vi "MPS_ErrorMessage.vi"(11 "error code (no error:0)":i32=5001) -> (0 "error out":errorcluster, 1 "message":string=" INSTRUCTIONS:\r\rNormal Use:  When using subVIs that incorporate the error in/error out (or error I/O) structure, place this handler where you want to inform the user of an error, typically at the end of the I/O data path, as the last action of the program.  If the error in error? is ERROR, the handler creates a message describing the error and its source.  If the type of dialog = 1 (default), the message is displayed to the user, who can only acknowedge it.  If the type = 2, the user can acknowledge the message or abort execution; aborting a program with active I/O is not recommended.  If the type = 0, no message is displayed; this is used to process the error programmatically, and the error out cluster elements are wired to individual terminals for that reason.  \r\rOther Use:\n\r\nlocal testing.  To test the error code of a subVI or function that does not have the error I/O structure, you can wire its error code and a source string to the local error code and error source inputs.  If error in error? indicates no error and error code is not equal to 0, the local code and source are substituted for the error in values, and error? is set TRUE (ERROR).", 3 "code out":i32 format="%0.0f", 5 "error?":bool)   [LabVIEW 2021]
uses:
  <vilib>/Utility/error.llb/DialogType.ctl
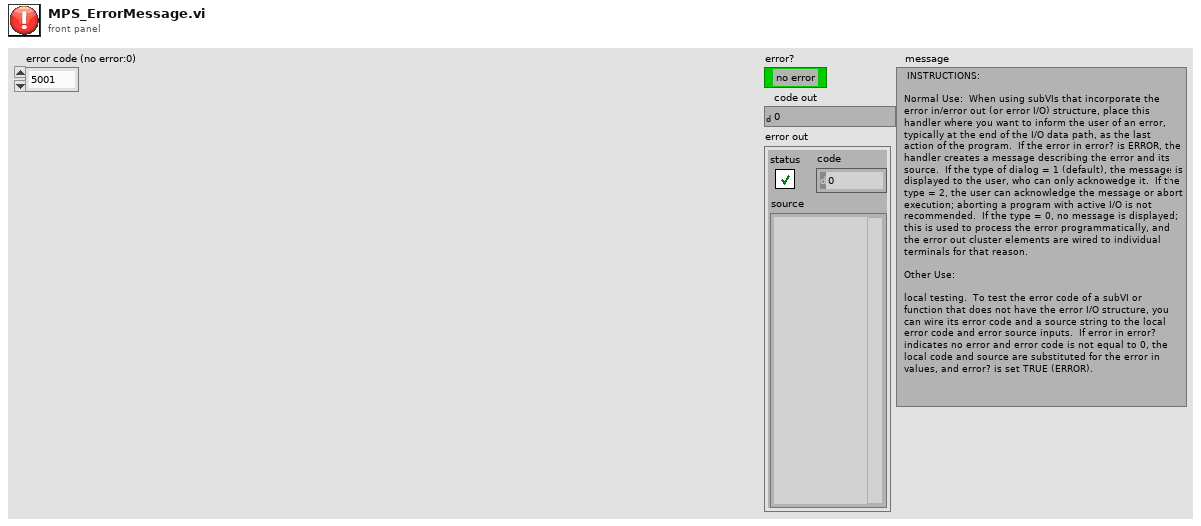
[diagram p1: front panel]
types:
  T1 = typedef "DialogType.ctl" = u16
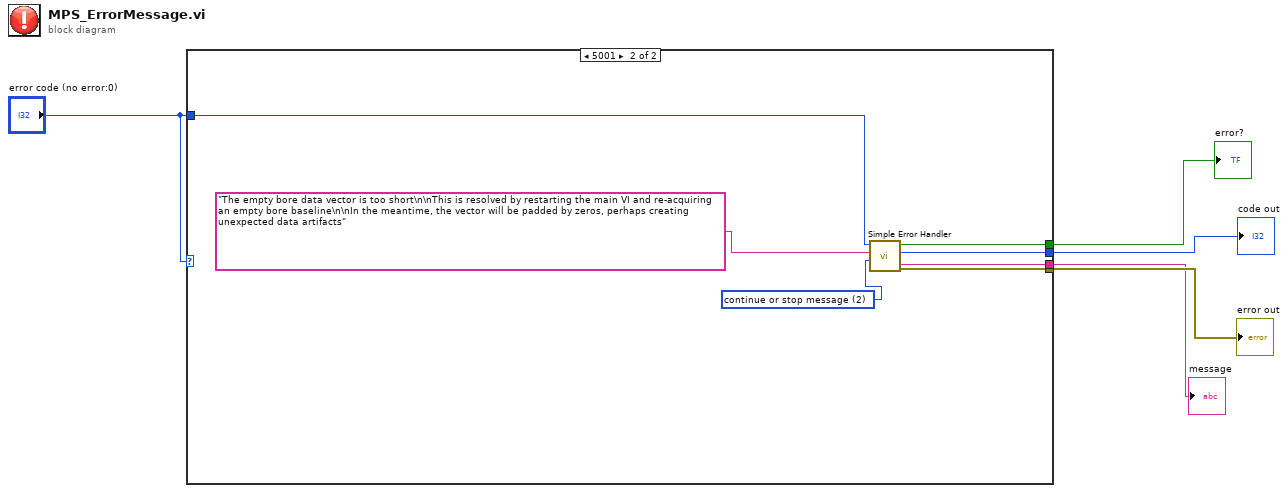
[diagram p0: block diagram]
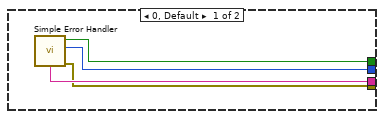
[diagram p2: hidden frame]
diagram:
  n1 = case shown="5001" "error code (no error:0)" {
    tunnel: "error code (no error:0)" -> [_ w16]
    tunnel: [w9 w13] -> w5
    tunnel: [w8 w12] -> w4
    tunnel: [w6 w11] -> w3
    tunnel: [w7 w10] -> w2
    frame 0, Default {
      n2 = call <vilib>:"Simple Error Handler.vi"() -> ("error?"=w9:bool, "code out"=w8:i32, "error out"=w6:errorcluster, "message"=w7:string)  [unwired: 5 in, 1 out]
    }
    frame 5001 {
      w14 = T1 2 items=["no dialog", "OK message", "continue or stop message", "OK message + warnings", "continue/stop + warnings"] ("type of dialog (OK msg:1)")
      n3 = call <vilib>:"Simple Error Handler.vi"("error code (no error:0)"=w16, "error source (\" \")"="The empty bore data vector is too short\n\nThis is resolved by restarting the main VI and re-acquiring an empty bore baseline\n\nIn the meantime, the vector will be padded by zeros, perhaps creating unexpected data artifacts" ("error source (\" \")"), "type of dialog (OK msg:1)"=w14) -> ("error?"=w13:bool, "code out"=w12:i32, "error out"=w11:errorcluster, "message"=w10:string)  [unwired: 2 in, 1 out]
    }
  }
  "error?" <- w5
  "code out" <- w4
  "error out" <- w3
  "message" <- w2
